vi "LC2_main.vi"() -> ()   [LabVIEW 2016]
uses:
  LC2_Global.vi
  Communication/Global communication output.vi
  LabVIEW Data/MathScriptVIs/MCStatic_36913153632_2bc289e0a5f717e12810d9cf21ccd4a4.vi
  <instcachedir>/0/MCStatic_36913153632_2bc289e0a5f717e12810d9cf21ccd4a4_D477B428622C441095E26A127D1E036B.lvgen/MCStatic_36913153632_2bc289e0a5f717e12810d9cf21ccd4a4_D477B428622C441095E26A127D1E036B_000.vi
  <vilib>/imath/engines/lvmath2/RunTimeEngine/BuiltInFunctions/abs/NIMS_abs(signed).vi
  <instcachedir>/0/NIMS_abs(signed)_C4FCB8E6058B49B797C7C8D53CA5F6EC.lvgen/NIMS_abs(signed)_C4FCB8E6058B49B797C7C8D53CA5F6EC_000.vi
  <vilib>/imath/engines/lvmath2/RunTimeEngine/NodeEndStatement/NIMS_NodeEndStatement_Output.vi
  <instcachedir>/0/NIMS_NodeEndStatement_Output_53EC0D466D134D7ABD903AC30B43404B.lvgen/NIMS_NodeEndStatement_Output_53EC0D466D134D7ABD903AC30B43404B_001.vi
  <vilib>/imath/engines/lvmath2/RunTimeEngine/ErrorHandling/NIMS_Finalize Error.vi
  BESS_LC/PIcontroller.m
panel:
  in  "p_in":dbl=0.2
  in  "i_in":dbl=0.2
  in  "p_an":dbl
  in  "i_an":dbl=0.01
  out "error out":errorcluster
  in  "Enable":bool=TRUE
  in  "i_mag":dbl=0.1
  in  "p_mag":dbl=0.1
  out "MGCC_to_BESS":dbl[](array[numeric])=[1.0, 0.0, 0.0, 3.563228138753649, -0.018765661995147957, 6.679101716144942e-12, 1.8051253380946264e-08, -2.7375026689924198e-09, 0.0, 0.0, 0.0, 0.0, 0.0, 0.0, 0.0, 0.0, 0.0, 0.0, 0.0, 0.0, 0.0, 0.0] format="%#_6f"
  out "Waveform Chart 2":dbl(graph)=-1.8051253380946264e-08
  out "Waveform Chart":dbl[][](graph)=[[-2.7375026689924198e-09, 3.5632281387562528, -6.679101716144942e-12]]
  # "Copyright <2020> <The University of Tennessee at Knoxville and the University of Tennessee Research Foundation>\n\nRedistribution and use in source and binary forms, with or without modification, are permitted provided that the following conditions are met:\n\n1. Redistributions of source code must retain the above copyright notice, this list of conditions and the following disclaimer.\n\n2. Redistributions in binary form must reproduce the above copyright notice, this list of conditions and the following disclaimer in the documentation and/or other materials provided with the distribution.\n\n3. Neither the name of the copyright holder nor the names of its contributors may be used to endorse or promote products derived from this software without specific prior written permission.\n\nTHIS SOFTWARE IS PROVIDED BY THE COPYRIGHT HOLDERS AND CONTRIBUTORS \"AS IS\" AND ANY EXPRESS OR IMPLIED WARRANTIES, INCLUDING, BUT NOT LIMITED TO, THE IMPLIED WARRANTIES OF MERCHANTABILITY AND FITNESS FOR A PARTICULAR PURPOSE ARE DISCLAIMED. IN NO EVENT SHALL THE COPYRIGHT HOLDER OR CONTRIBUTORS BE LIABLE FOR ANY DIRECT, INDIRECT, INCIDENTAL, SPECIAL, EXEMPLARY, OR CONSEQUENTIAL DAMAGES (INCLUDING, BUT NOT LIMITED TO, PROCUREMENT OF SUBSTITUTE GOODS OR SERVICES; LOSS OF USE, DATA, OR PROFITS; OR BUSINESS INTERRUPTION) HOWEVER CAUSED AND ON ANY THEORY OF LIABILITY, WHETHER IN CONTRACT, STRICT LIABILITY, OR TORT (INCLUDING NEGLIGENCE OR OTHERWISE) ARISING IN ANY WAY OUT OF THE USE OF THIS SOFTWARE, EVEN IF ADVISED OF THE POSSIBILITY OF SUCH DAMAGE."
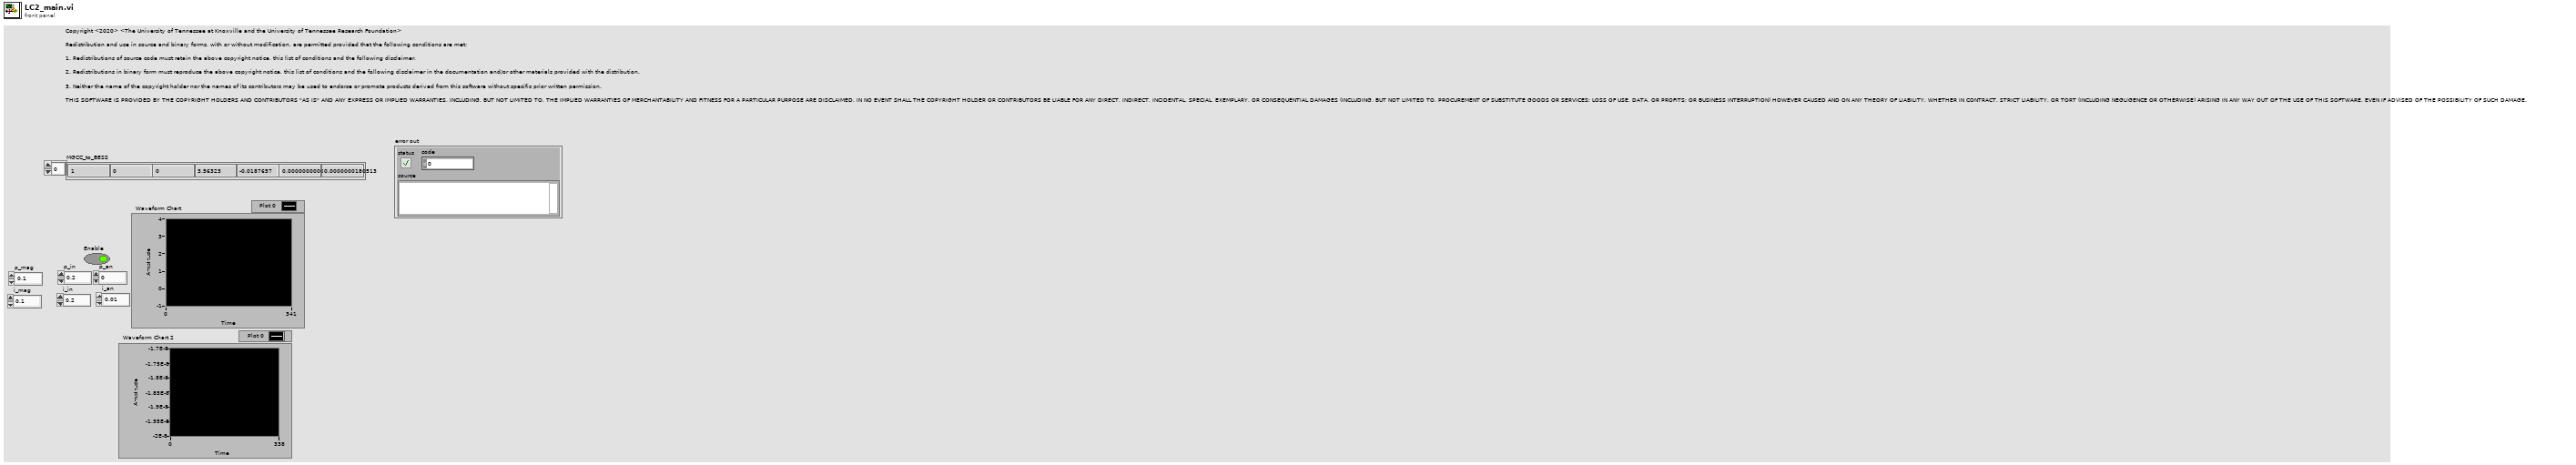
[diagram p1: front panel]
types:
  T1 = typedef "NI_Matrix.lvlib/RealMatrix.ctl" = dbl[][]
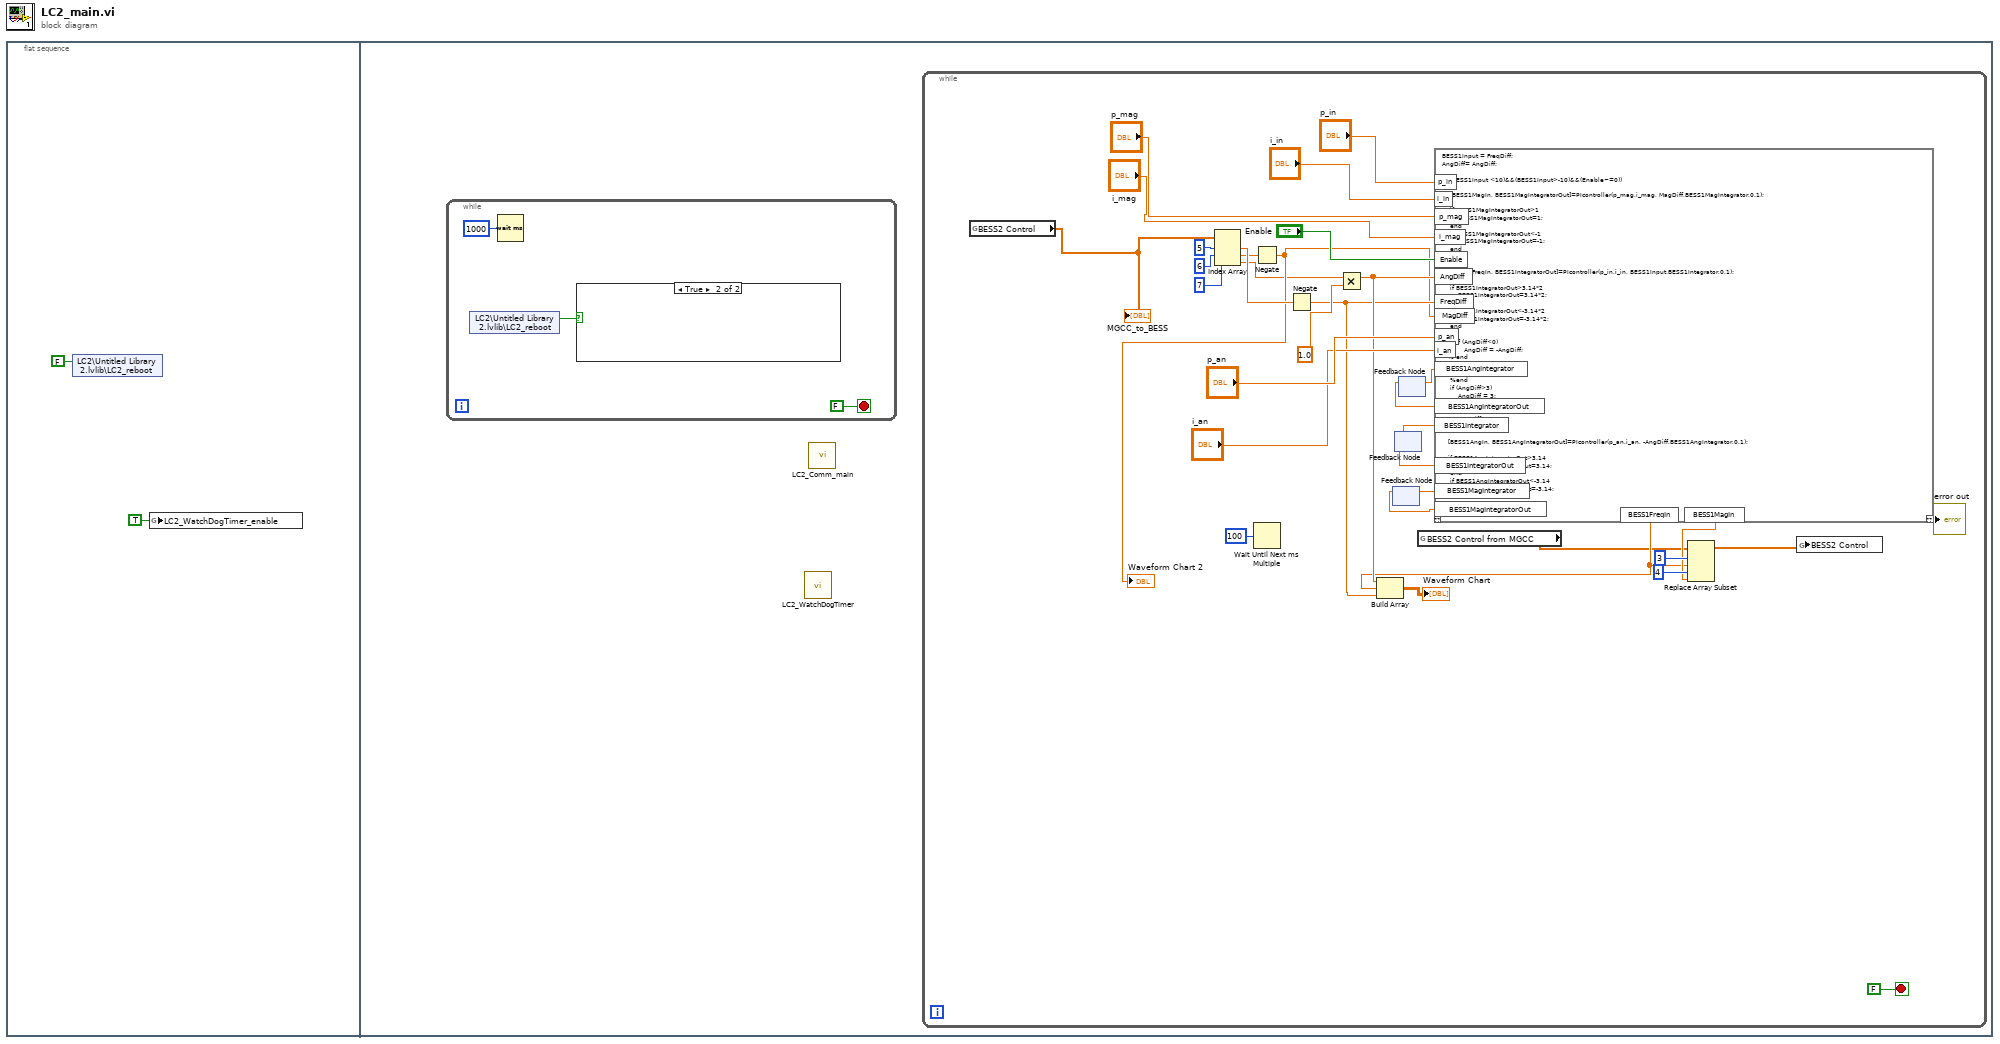
[diagram p0: block diagram]
diagram:
  n1 = flat-sequence {
    frame #0 {
      n2 = shared-variable "LC2\\Untitled Library 2.lvlib\\LC2_reboot"(FALSE ("LC2_reboot")) -> ()  [unwired: 1 in, 1 out]
      n3 = global write "LC2_Global.vi" "LC2_WatchDogTimer_enable"(TRUE ("LC2_WatchDogTimer_enable")) -> ()
    }
    frame #1 {
      n4 = while {
        stop <- FALSE stop-if-true
        n5 = shared-variable "LC2\\Untitled Library 2.lvlib\\LC2_reboot"() -> (w3:bool)  [unwired: 1 in, 1 out]
        n6 = Wait (ms)(milliseconds to wait=u32 1000) -> ()  [unwired: 1 out]
        n7 = case shown="True" w3 {
          frame False {
          }
          frame True {
          }
        }
      }
      n8 = call "LC2_WatchDogTimer.vi"() -> ()  [unwired: 12 in]
      n9 = call "LC2_Comm_main.vi"() -> ()  [unwired: 12 in]
      n10 = while {
        stop <- FALSE stop-if-true
        n11 = global read "Global communication output.vi" "BESS2 Control"() -> (w13:dbl[])
        "MGCC_to_BESS" <- w13
        n12 = Index Array(array=w13, index #1=5 ("index"), index #2=6 ("index"), index #3=7 ("index")) -> (element #1=w10:dbl, element #2=w9:dbl, element #3=w6:dbl)
        n13 = Negate(x=w9) -> (-x=w7:dbl)
        "Waveform Chart 2" <- w7
        n14 = Wait Until Next ms Multiple(millisecond multiple=u32 100) -> ()  [unwired: 1 out]
        n15 = Negate(x=w10) -> (-x=w8:dbl)
        n16 = Multiply(x=w6, y=1.0) -> (x*y=w18:dbl)
        n17 = feedback #1() -> (w20:dbl)  [unwired: 1 in]
        n18 = feedback #2() -> (w38:dbl)  [unwired: 1 in]
        n19 = feedback #3() -> (w35:dbl)  [unwired: 1 in]
        n20 = global read "Global communication output.vi" "BESS2 Control from MGCC"() -> (w12:dbl[])
        n21 = mathscript code="BESS1Input = FreqDiff;\nAngDiff= AngDiff;\n\nif ((BESS1Input <10)&&(BESS1Input>-10)&&(Enable~=0))\n\n    [BESS1MagIn, BESS1MagIntegratorOut]=PIcontroller(p_mag,i_mag, MagDiff,BESS1MagIntegrator,0.1);\n   \n    if BESS1MagIntegratorOut>1\n        BESS1MagIntegratorOut=1;\n    end\n    if BESS1MagIntegratorOut<-1\n        BESS1MagIntegratorOut=-1;\n    end\n\n\n    [BESS1FreqIn, BESS1IntegratorOut]=PIcontroller(p_in,i_in, BESS1Input,BESS1Integrator,0.1);\n   \n    if BESS1IntegratorOut>3.14*2\n        BESS1IntegratorOut=3.14*2;\n    end\n    if BESS1IntegratorOut<-3.14*2\n        BESS1IntegratorOut=-3.14*2;\n    end\n\n%    if (AngDiff<0)\n %       AngDiff = -AngDiff;\n   % end \n    %if (AngDiff> 5)\n     %   AngDiff = 0;\n    %end \n    if (AngDiff>3)\n        AngDiff = 3;\n    end \n    if (AngDiff<-3)\n        AngDiff = -3;\n    end \n\n   [BESS1AngIn, BESS1AngIntegratorOut]=PIcontroller(p_an,i_an, -AngDiff,BESS1AngIntegrator,0.1);\n\n   if BESS1AngIntegratorOut>3.14\n        BESS1AngIntegratorOut=3.14;\n    end\n    if BESS1AngIntegratorOut<-3.14\n        BESS1AngIntegratorOut=-3.14;\n    end\n    \n    if abs(FreqDiff)<0.2\n        BESS1FreqIn = BESS1FreqIn + BESS1AngIn;\n    else\n        BESS1AngIntegratorOut = 0;\n    end\n    if (BESS1FreqIn > 3.14*2) \n          BESS1FreqIn = 3.14*2;\n    end\n    if (BESS1FreqIn < -3.14*2) \n          BESS1FreqIn = -3.14*2;\n    end\n\n    if (AngDiff ==0)&&(FreqDiff == 0) && (MagDiff== 0)\n        BESS1FreqIn = 0;\n        BESS1MagIn = 0;\n        BESS1IntegratorOut = 0;\n        BESS1MagIntegratorOut = 0;\n        BESS1AngIntegratorOut = 0;\n    end\n\nelse\nBESS1FreqIn = 0;\nBESS1MagIn = 0;\nBESS1IntegratorOut = 0;\nBESS1MagIntegratorOut = 0;\nBESS1AngIntegratorOut = 0;\nend"("AngDiff"=w18, "BESS1Integrator"=w38, "FreqDiff"=w8, "BESS1AngIntegrator"=w35, "Enable"="Enable", "p_in"="p_in", "i_in"="i_in", "p_an"="p_an", "i_an"="i_an", "p_mag"="p_mag", "i_mag"="i_mag", "BESS1MagIntegrator"=w20, "MagDiff"=w7) -> ("??"=→"error out":errorcluster, "BESS1IntegratorOut"=w37:dbl, "BESS1FreqIn"=w14:dbl, "BESS1AngIntegratorOut"=w36:dbl, "BESS1MagIntegratorOut"=w21:dbl, "BESS1MagIn"=w15:dbl)  [unwired: 1 in]
        n22 = Build Array(w18, w14, w8) -> (→"Waveform Chart":T1)
        n23 = feedback-in #1(w21) -> ()
        n24 = feedback-in #2(w37) -> ()
        n25 = feedback-in #3(w36) -> ()
        n26 = Replace Array Subset(array=w12, new element #1=w14, index #1=3 ("index"), new element #2=w15, index #2=4 ("index")) -> (w11:dbl[])
        n27 = global write "Global communication output.vi" "BESS2 Control"(w11) -> ()
      }
    }
  }
